vi "Load_tracker_settings.vi"(0 "PORT NAME":string="Inlet_Heaters") -> ()   [LabVIEW 2011]
uses:
  Anemometry/Anemometry Sub Vis/Globals/Constants_global.vi
panel:
  out "Number of Locations Changed":i32
  in  "MODULE ADDRESS":i32=1
  out "Locations Edited":string[](array[string])
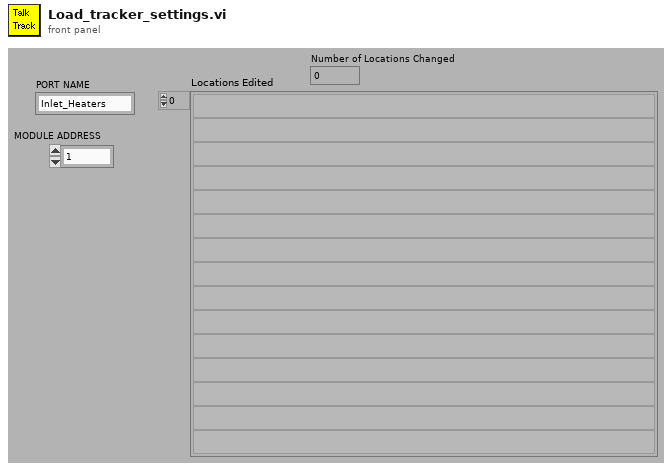
[diagram p1: front panel]
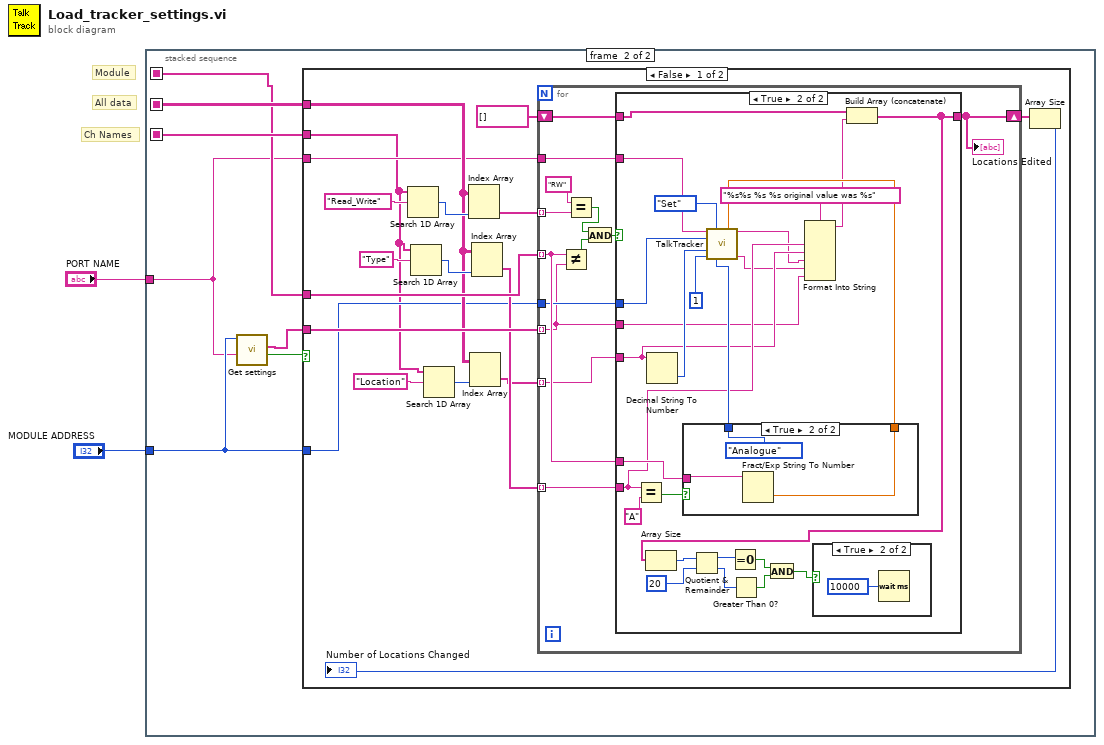
[diagram p0: block diagram]
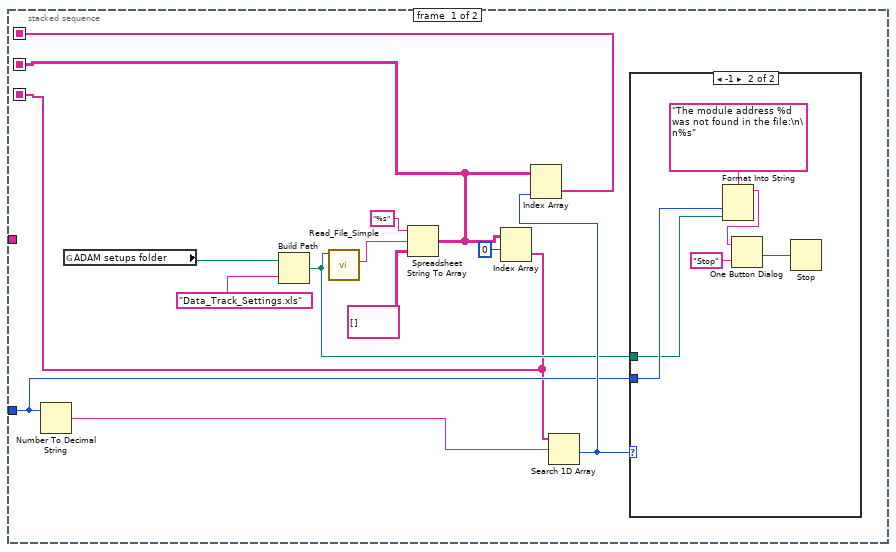
[diagram p2: hidden frame]
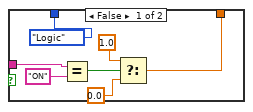
[diagram p6: hidden frame]
diagram:
  # "Ch Names"
  # "All data"
  # "Module"
  n1 = stacked-sequence {
    seq-local: [w3 _] -> [_ w25]
    seq-local: [w5 _] -> [_ w26]
    seq-local: [w4 _] -> [_ w27]
    tunnel: "MODULE ADDRESS" -> [w7 w23]
    tunnel: "PORT NAME" -> [_ w22]
    frame #0 {
      n2 = Number To Decimal String(number=w7) -> (decimal integer string=w9:string)  [unwired: 1 in]
      n3 = global read "Constants_global.vi" "ADAM setups folder"() -> (w12:path)
      n4 = Build Path(base path=w12, name or relative path="Data_Track_Settings.xls") -> (appended path=w6:path)
      n5 = call "Read_File_Simple.vi"("Filename"=w6) -> ("string"=w15:string)  [unwired: 4 in, 5 out]
      n6 = Spreadsheet String To Array(format string="%s", spreadsheet string=w15, array type (2D Dbl)=string[][] []) -> (array=w5:string[][])  [unwired: 1 in]
      n7 = Index Array(array=w5, index (row)=0) -> (element=w4:string[])  [unwired: 1 in]
      n8 = Search 1D Array(1D array=w4, element=w9) -> (index of element=w8:i32)  [unwired: 1 in]
      n9 = Index Array(array=w5, index (col)=w8) -> (element=w3:string[])  [unwired: 1 in]
      n10 = case shown="-1" w8 {
        tunnel: w7 -> [_ w18]
        tunnel: w6 -> [_ w17]
        frame 0, Default {
        }
        frame -1 {
          n11 = Format Into String(format string="The module address %d was not found in the file:\n\n%s" ("message"), w18, w17) -> (resulting string=w16:string)  [unwired: 2 in, 1 out]
          n12 = One Button Dialog(message=w16, button name ("OK")="Stop") -> (true=w20:bool)
          n13 = Stop(stop? (T)=w20) -> ()
        }
      }
    }
    frame #1 {
      n14 = call "Get settings.vi"("MODULE ADDRESS"=w23, "PORT NAME"=w22) -> ("Settings"=w24:string[], "Error"=w28:bool)  [unwired: 6 in, 1 out]
      n15 = case shown="False" w28 {
        tunnel: w27 -> [w29 _]
        tunnel: w26 -> [w36 _]
        tunnel: w25 -> [w41 _]
        tunnel: w24 -> [w40 _]
        tunnel: w23 -> [w34 _]
        tunnel: w22 -> [w33 _]
        frame False {
          n16 = Search 1D Array(1D array=w29, element="Read_Write") -> (index of element=w45:i32)  [unwired: 1 in]
          n17 = Search 1D Array(1D array=w29, element="Type") -> (index of element=w44:i32)  [unwired: 1 in]
          n18 = Search 1D Array(1D array=w29, element="Location") -> (index of element=w37:i32)  [unwired: 1 in]
          n19 = Index Array(array=w36, index (col)=w45) -> (element=w42:string[])  [unwired: 1 in]
          n20 = Index Array(array=w36, index (col)=w37) -> (element=w35:string[])  [unwired: 1 in]
          n21 = Index Array(array=w36, index (col)=w44) -> (element=w39:string[])  [unwired: 1 in]
          n22 = for {
            tunnel: w42 -> [w59] mode=indexing
            tunnel: w41 -> [w53] mode=indexing
            tunnel: w40 -> [w47] mode=indexing
            tunnel: w39 -> [w54] mode=indexing
            tunnel: w35 -> [w52] mode=indexing
            tunnel: w34 -> [w51]
            tunnel: w33 -> [w50]
            shift-right: [w48] -> w31
            shift-left: string[] [] -> [w49]
            n23 = Not Equal?(x=w53, y=w47) -> (x != y?=w56:bool)
            n24 = Equal?(x="RW", y=w59) -> (x = y?=w57:bool)
            n25 = And(x=w57, y=w56) -> (x .and. y?=w55:bool)
            n26 = case shown="True" w55 {
              tunnel: w54 -> [_ w75]
              tunnel: w53 -> [_ w84]
              tunnel: w52 -> [_ w74]
              tunnel: w51 -> [_ w79]
              tunnel: w50 -> [_ w78]
              tunnel: [w60 w62] -> w48
              tunnel: w49 -> [w60 w76]
              tunnel: w47 -> [_ w61]
              frame False {
              }
              frame True {
                n27 = Equal?(x=w75, y="A") -> (x = y?=w85:bool)
                n28 = Decimal String To Number(string=w74) -> (number=w80:i32)  [unwired: 2 in, 1 out]
                n29 = case shown="True" w85 {
                  tunnel: w84 -> [w94 w96]
                  tunnel: [w89 w95] -> w83
                  tunnel: [enum16{"Logic", "Analogue"}."Logic" ("Analogue") enum16{"Logic", "Analogue"}."Analogue" ("Analogue")] -> w82
                  frame False {
                    n30 = Equal?(x=w94, y="ON") -> (x = y?=w92:bool)
                    n31 = Select(t=1.0, s=w92, f=0.0) -> (s? t:f=w89:dbl)
                  }
                  frame True {
                    n32 = Fract/Exp String To Number(string=w96) -> (number=w95:dbl)  [unwired: 3 in, 1 out]
                  }
                }
                n33 = call "TalkTracker.vi"("PORT NAME"=w78, "Set"=enum16{"Set", "Read"}."Set", "Value to set"=w83, "MODULE ADDRESS"=w79, "LOCATION"=w80, "NO. LOCATIONS"=1, "Analogue"=w82) -> ("Response"=w73:string, "Comment out"=w72:string)  [unwired: 6 in, 1 out]
                n34 = Format Into String(format string="%s%s %s %s original value was %s", w75, w74, w73, w72, w61) -> (resulting string=w70:string)  [unwired: 2 in, 1 out]
                n35 = Build Array (concatenate)(w76, w70) -> (w62:string[])
                n36 = Array Size(array=w62) -> (size(s)=w68:i32)
                n37 = Quotient & Remainder(x=w68, y=20) -> (x-y*floor(x/y)=w66:i32, floor(x/y)=w67:i32)
                n38 = Equal To 0?(x=w66) -> (x = 0?=w64:bool)
                n39 = Greater Than 0?(x=w67) -> (x > 0?=w65:bool)
                n40 = And(x=w64, y=w65) -> (x .and. y?=w63:bool)
                n41 = case shown="True" w63 {
                  frame False {
                  }
                  frame True {
                    n42 = Wait (ms)(milliseconds to wait=u32 10000) -> ()  [unwired: 1 out]
                  }
                }
              }
            }
            "Locations Edited" <- w48
          }
          n43 = Array Size(array=w31) -> (size(s)=→"Number of Locations Changed":i32)
        }
        frame True {
        }
      }
    }
  }
